vi "Increment Call Count.vi"(10 "Call in":refnum<class "VI Call.lvclass">, 11 "Expected Calls in":map{refnum<class "VI Call.lvclass">, i32}(c390)) -> (3 "Expected Calls out":map{refnum<class "VI Call.lvclass">, i32}(c390))   [LabVIEW 2020, in "One or More.lvclass"]
uses:
  One or More.lvclass
  Call/VI Call.lvclass
  <vilib>/Utility/miscctls.llb/LVMapReplaceAction.ctl
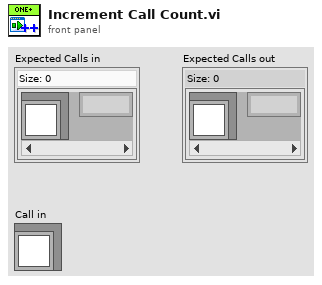
[diagram p1: front panel]
types:
  T1 = typedef "LVMapReplaceAction.ctl" = enum32{"Modify Entry only if found", "Add or Modify Entry", "Delete Entry"}
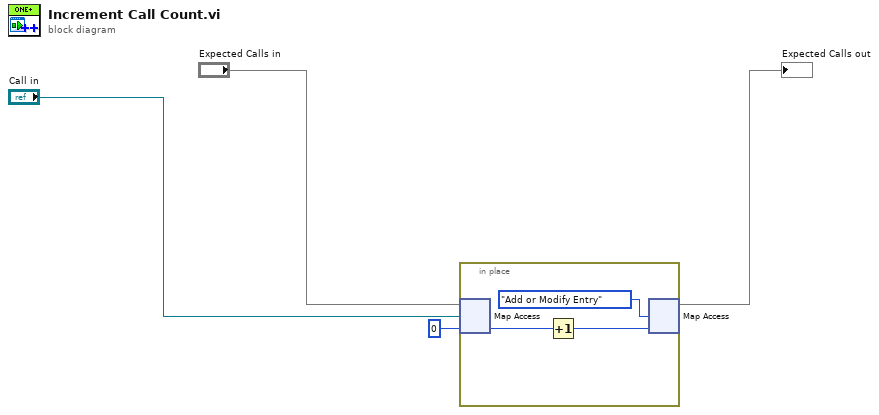
[diagram p0: block diagram]
diagram:
  n1 = in-place {
    n2 = in-place-map #1("Expected Calls in", "Call in", 0) -> (w7:i32)  [unwired: 1 out]
    n3 = Increment(x=w7) -> (x+1=w6:i32)
    n4 = in-place-map #1(w6, LVMapReplaceAction."Add or Modify Entry" ("action")) -> (→"Expected Calls out":map{refnum<class "VI Call.lvclass">, i32})  [unwired: 2 out]
  }
